vi "checkLBValue.vi"() -> (0 "LB new status":bool[](array[boolean]))   [LabVIEW 2012]
uses:
  <vilib>/Instr/_visa.llb/Select Event Type.ctl
  GlobalArduino.vi
  GlobalLB.vi
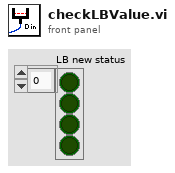
[diagram p1: front panel]
types:
  T1 = typedef "Select Event Type.ctl" = u32
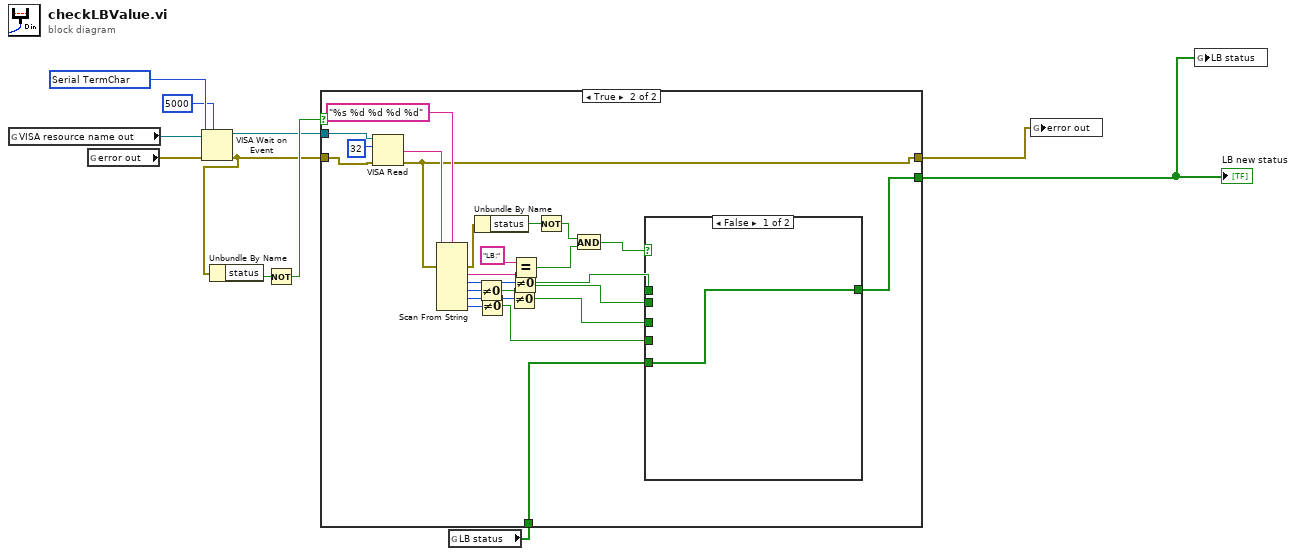
[diagram p0: block diagram]
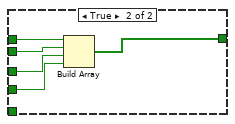
[diagram p3: hidden frame]
diagram:
  w6 = T1 1073684516 items=["Service Request"=1073684491, "Trigger"=3221168138, "Clear"=1073684493, "VXI Signal"=1073684512, "VXI/VME Interrupt"=3221168161, "VXI/VME Sysfail"=1073684509, "VXI/VME Sysreset"=1073684510, "GPIB CIC"=1073684498, "GPIB Talk"=1073684499, "GPIB Listen"=1073684500, "PXI Interrupt"=1073684514, "Serial Break"=1073684515, "Serial TermChar"=1073684516, "Serial CTS"=1073684521, "Serial DSR"=1073684522, "Serial DCD"=1073684524, "Serial RI"=1073684526, "Serial Character"=1073684533, "USB Interrupt"=1073684535, "All Enabled"=1073709055] ("Event Type")
  n1 = global read "GlobalArduino.vi" "VISA resource name out"() -> (w11:refnum<visa-resource-name>)
  n2 = global read "GlobalArduino.vi" "error out"() -> (w10:errorcluster)
  n3 = VISA Wait on Event(7:u32 5000 ("timeout (0)"), 8:w10, 10:w6, 11:w11) -> (0:w2:errorcluster, 3:w7:refnum<visa-resource-name>)  [unwired: 1 in, 2 out]
  n4 = Unbundle By Name(w2) -> ("status"=w9:bool)
  n5 = Not(x=w9) -> (.not. x?=w8:bool)
  n6 = global read "GlobalLB.vi" "LB status"() -> (w4:bool[])
  n7 = case shown="True" w8 {
    tunnel: w7 -> [_ w35]
    tunnel: w4 -> [w13 w30]
    tunnel: [w13 w22] -> w5
    tunnel: w2 -> [w12 w15]
    tunnel: [w12 w14] -> w1
    frame False {
    }
    frame True {
      n8 = VISA Read(VISA resource name=w35, byte count=u32 32, error in (no error)=w15) -> (read buffer=w34:string, error out=w14:errorcluster)  [unwired: 2 out]
      n9 = Scan From String(format string="%s %d %d %d %d", input string=w34, error in=w14) -> (error out=w29:errorcluster, output 1=w32:string, output 2=w28:i32, output 3=w27:i32, output 4=w21:i32, output 5=w20:i32)  [unwired: 6 in, 2 out]
      n10 = Unbundle By Name(w29) -> ("status"=w26:bool)
      n11 = Not Equal To 0?(x=w27) -> (x != 0?=w18:bool)
      n12 = Not Equal To 0?(x=w20) -> (x != 0?=w16:bool)
      n13 = Not Equal To 0?(x=w21) -> (x != 0?=w17:bool)
      n14 = Not Equal To 0?(x=w28) -> (x != 0?=w19:bool)
      n15 = Equal?(x="LB:", y=w32) -> (x = y?=w24:bool)
      n16 = Not(x=w26) -> (.not. x?=w25:bool)
      n17 = And(x=w25, y=w24) -> (x .and. y?=w23:bool)
      n18 = case shown="False" w23 {
        tunnel: [w37 w38] -> w22
        tunnel: w30 -> [w37 _]
        tunnel: w19 -> [_ w42]
        tunnel: w18 -> [_ w41]
        tunnel: w17 -> [_ w40]
        tunnel: w16 -> [_ w39]
        frame False {
        }
        frame True {
          n19 = Build Array(w42, w41, w40, w39) -> (w38:bool[])
        }
      }
    }
  }
  "LB new status" <- w5
  n20 = global write "GlobalArduino.vi" "error out"(w1) -> ()
  n21 = global write "GlobalLB.vi" "LB status"(w5) -> ()
